vi "RunAllTests.vi"() -> ()   [LabVIEW 2019]
panel:
  out "Ramsete":bool
  out "Profiled PID":bool
  out "Twist":bool
  out "Translation":bool
  out "Transform":bool
  out "Rotation":bool
  out "Pose":bool
  out "Median Filter":bool
  out "Cubic Spline":bool
  out "Linear System ID":bool
  out "Kalman filter test":bool
  out "Discretization 2":bool
  out "PID tolerance":bool
  out "PID Input / Output Tests Passed":bool
  out "LQR Passed":bool
  out "Diff Drive Kinematics Passed":bool
  out "Angle Stats Passed":bool
  # "cubic spline"
  # "Ramsete"
  # "Angle Statistics"
  # "median filter"
  # "Diff Drive Kine"
  # "Linear Quadratic Regulator"
  # "Pose"
  # "PID Input / Output"
  # "Rotation"
  # "Transform\nMAY NOT BE DONE"
  # "PID tolerance"
  # "Discretization"
  # "Translation"
  # "Kalman Filter Test"
  # "Twist"
  # "Linear System ID"
  # "Profiled PID"
  # "Diff Drive Odom"
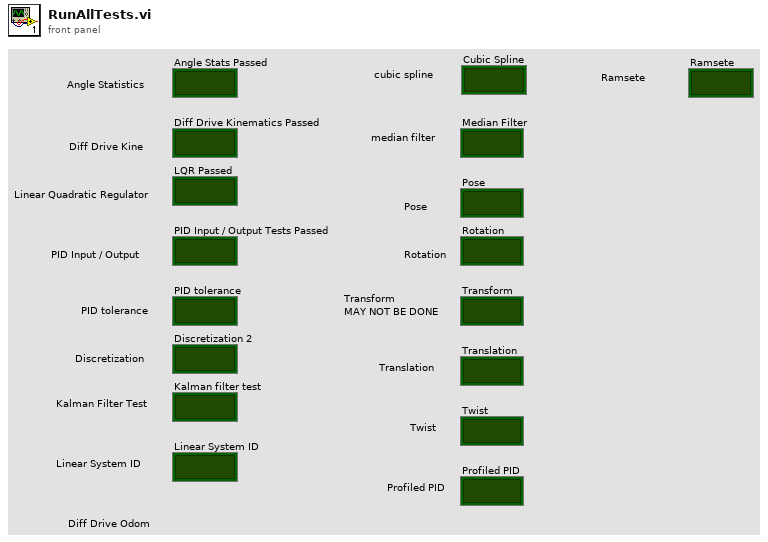
[diagram p1: front panel]
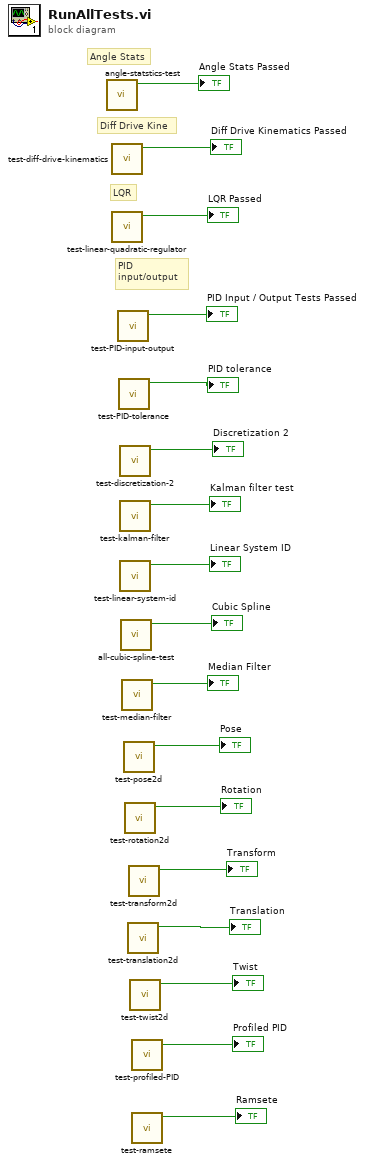
[diagram p0: block diagram]
diagram:
  # "PID\ninput/output"
  # "LQR"
  # "Diff Drive Kine"
  # "Angle Stats"
  n1 = call "angle-statstics-test.vi"() -> ("All Passed"=→"Angle Stats Passed":bool)  [unwired: 11 in]
  n2 = call "test-diff-drive-kinematics.vi"() -> ("All Passed"=→"Diff Drive Kinematics Passed":bool)  [unwired: 11 in]
  n3 = call "test-linear-quadratic-regulator.vi"() -> ("ALL TESTS GOOD"=→"LQR Passed":bool)  [unwired: 11 in]
  n4 = call "test-PID-input-output.vi"() -> ("All Passed"=→"PID Input / Output Tests Passed":bool)  [unwired: 11 in]
  n5 = call "test-PID-tolerance.vi"() -> ("All Tests Passed"=→"PID tolerance":bool)  [unwired: 11 in]
  n6 = call "test-discretization-2.vi"() -> ("All Tests Passed"=→"Discretization 2":bool)  [unwired: 11 in]
  n7 = call "test-kalman-filter.vi"() -> ("ALL TESTS PASSED"=→"Kalman filter test":bool)  [unwired: 11 in]
  n8 = call "test-linear-system-id.vi"() -> ("All tests passed"=→"Linear System ID":bool)  [unwired: 11 in]
  n9 = call "all-cubic-spline-test.vi"() -> ("ALL TESTS PASSED"=→"Cubic Spline":bool)  [unwired: 11 in]
  n10 = call "test-median-filter.vi"() -> ("ALL TESTS PASSED"=→"Median Filter":bool)  [unwired: 11 in]
  n11 = call "test-pose2d.vi"() -> ("All PASSED"=→"Pose":bool)  [unwired: 11 in]
  n12 = call "test-rotation2d.vi"() -> ("ALL TESTS PASSED"=→"Rotation":bool)  [unwired: 11 in]
  n13 = call "test-translation2d.vi"() -> ("All PASSED"=→"Translation":bool)  [unwired: 11 in]
  n14 = call "test-transform2d.vi"() -> ("All PASSED"=→"Transform":bool)  [unwired: 11 in]
  n15 = call "test-twist2d.vi"() -> ("All PASSED"=→"Twist":bool)  [unwired: 11 in]
  n16 = call "test-profiled-PID.vi"() -> ("Test Passed 0"=→"Profiled PID":bool)  [unwired: 11 in]
  n17 = call "test-ramsete.vi"() -> ("AtReference End"=→"Ramsete":bool)  [unwired: 11 in]
